vi "PH_BeamlineController.Path set Source.vi"(0 "i ref in":refnum<vi>, 5 "error in (no error)":errorcluster) -> (14 "i ref out":refnum<vi>, 17 "Path changed?":bool, 19 "error out":errorcluster)   [LabVIEW 2014, in "PH_BeamlineController.lvlib"]
doc: "This VI writes incoming Information to own Attributes if the new value differs from the stored."
uses:
  PH_BeamlineController.lvlib
  PH_BeamlineController.Sources.ctl
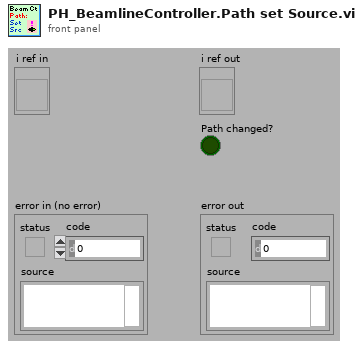
[diagram p1: front panel]
types:
  T1 = typedef "PH_BeamlineController.lvlib/PH_BeamlineController.Sources.ctl" = enum16{"None", "YLF", "fs-Frontend", "ns-Frontend", "YLF and ns-Frontend", "fs- and ns-Frontend"}
  T2 = typedef "PH_BeamlineController.lvlib/PH_BeamlineController.Source Attributes.ctl" = cluster{"Name":T1, "GUI Ref":refnum<vi>, "Current State":bool, "Wanted State":bool}
  T3 = typedef "PH_BeamlineController.lvlib/PH_BeamlineController.i attribute.ctl" = cluster{"Vacuum Exp LB":cluster{"Channel":string, "Limit [mbar]":dbl, "Pressure [mbar]":dbl, "GUI Ref":refnum<vi>}, "Sources":T2[], "PA DP Targets":T4[], "Path":cluster{"Source":T1, "PA DP Target":T5, "Target":T6}, "Targets":cluster{"Name":T6, "GUI Ref":refnum<vi>, "Current State":bool, "Wanted State":bool, "Enabled":bool}[], "Status Tags":cluster{"Name":string, "Status":T7}[], "special GUI Refs":T8}
  T4 = typedef "PH_BeamlineController.lvlib/PH_BeamlineController.PA DP Target Attributes.ctl" = cluster{"Name":T5, "GUI Ref":refnum<vi>, "Current State":bool, "Wanted State":bool, "Enabled":bool}
  T5 = typedef "PH_BeamlineController.lvlib/PH_BeamlineController.PA DP Targets.ctl" = enum16{"None", "Dump PA Delayed Beam", "Dump PA Undelayed Beam", "Dumps PA Delayed and Undelayed Beam"}
  T6 = typedef "PH_BeamlineController.lvlib/PH_BeamlineController.Targets.ctl" = enum16{"None", "PreAmp", "Dump Exp Laserlab", "Exp Laserlab", "Calorimeter", "Dump Exp Laserbay", "Exp Laserbay", "Dump Exp Z6", "Exp Z6"}
  T7 = typedef "PH_StatusHandler.lvlib/PH_StatusHandler.Status.ctl" = i16
  T8 = typedef "PH_BeamlineController.lvlib/PH_BeamlineController.special GUI Refs.ctl" = cluster{"PA-Backreflection-Meas":refnum<vi>, "fs_Synchrolock_Watch":refnum<vi>}
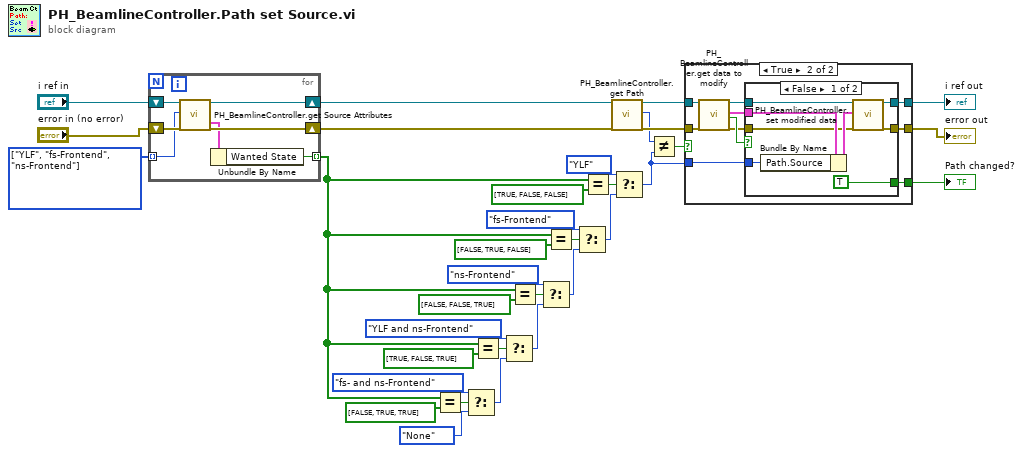
[diagram p0: block diagram]
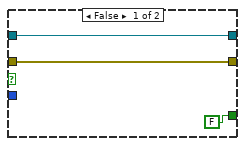
[diagram p2: hidden frame]
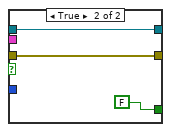
[diagram p3: hidden frame]
diagram:
  w24 = T1[] [enum."YLF", enum."fs-Frontend", enum."ns-Frontend"] items=["None", "YLF", "fs-Frontend", "ns-Frontend", "YLF and ns-Frontend", "fs- and ns-Frontend"]
  n1 = for {
    shift-right: [w40] -> w28
    shift-left: "error in (no error)" -> [w41]
    shift-right: [w38] -> w30
    shift-left: "i ref in" -> [w39]
    tunnel: [w36] -> w5 mode=indexing
    tunnel: w24 -> [w35] mode=indexing
    n2 = call "PH_BeamlineController.get Source Attributes.vi"("VI in"=w39, "Source"=w35, "error in (no error)"=w41) -> ("VI out"=w38:refnum<vi>, "Source Attributes"=w37:T2, "error out"=w40:errorcluster)  [unwired: 13 in, 1 out]
    n3 = Unbundle By Name(w37) -> ("Wanted State"=w36:bool)
  }
  n4 = Equal?(x=w5, y=bool[] [FALSE, TRUE, TRUE]) -> (x = y?=w7:bool)
  n5 = Select(t=PH_BeamlineController.Sources."fs- and ns-Frontend" ("Path.Source"), s=w7, f=PH_BeamlineController.Sources."None" ("Path.Source")) -> (s? t:f=w4:T1)
  n6 = Equal?(x=w5, y=bool[] [TRUE, FALSE, TRUE]) -> (x = y?=w11:bool)
  n7 = Select(t=PH_BeamlineController.Sources."YLF and ns-Frontend" ("Path.Source"), s=w11, f=w4) -> (s? t:f=w9:T1)
  n8 = Equal?(x=w5, y=bool[] [FALSE, FALSE, TRUE]) -> (x = y?=w15:bool)
  n9 = Select(t=PH_BeamlineController.Sources."ns-Frontend" ("Path.Source"), s=w15, f=w9) -> (s? t:f=w13:T1)
  n10 = Equal?(x=w5, y=bool[] [FALSE, TRUE, FALSE]) -> (x = y?=w19:bool)
  n11 = Select(t=PH_BeamlineController.Sources."fs-Frontend" ("Path.Source"), s=w19, f=w13) -> (s? t:f=w18:T1)
  n12 = Equal?(x=w5, y=bool[] [TRUE, FALSE, FALSE]) -> (x = y?=w22:bool)
  n13 = call "PH_BeamlineController.get Path.vi"("VI in"=w30, "error in (no error)"=w28) -> ("VI out"=w29:refnum<vi>, "Path: Source"=w1:T1, "error out"=w27:errorcluster)  [unwired: 12 in, 3 out]
  n14 = Select(t=PH_BeamlineController.Sources."YLF" ("Path.Source"), s=w22, f=w18) -> (s? t:f=w2:T1)
  n15 = Not Equal?(x=w1, y=w2) -> (x != y?=w31:bool)
  n16 = case shown="True" w31 {
    tunnel: w2 -> [_ w54]
    tunnel: [w44 w49] -> w33
    tunnel: [w43 w48] -> w34
    tunnel: w27 -> [w43 w47]
    tunnel: w29 -> [w44 w46]
    tunnel: [FALSE w45] -> w32
    frame False {
    }
    frame True {
      n17 = call "PH_BeamlineController.get data to modify.vi"("i ref in"=w46, "error in (no error)"=w47) -> ("i ref out"=w50:refnum<vi>, "i attribute"=w52:T3, "timed out"=w53:bool, "error out"=w51:errorcluster)  [unwired: 14 in]
      n18 = case shown="False" w53 {
        tunnel: w50 -> [w58 w65]
        tunnel: [w62 w65] -> w49
        tunnel: w51 -> [w57 w64]
        tunnel: [w61 w64] -> w48
        tunnel: w52 -> [w60 _]
        tunnel: w54 -> [w55 _]
        tunnel: [TRUE FALSE] -> w45
        frame False {
          n19 = Bundle By Name(cluster=w60, "Path.Source"=w55) -> (w59:T3)
          n20 = call "PH_BeamlineController.set modified data.vi"("i ref in"=w58, "i attribute"=w59, "error in (no error)"=w57) -> ("i ref out"=w62:refnum<vi>, "error out"=w61:errorcluster)  [unwired: 15 in]
        }
        frame True {
        }
      }
    }
  }
  "error out" <- w34
  "i ref out" <- w33
  "Path changed?" <- w32
